vi "Read Mail To Next Actor.vi"(8 "error in (no error)":errorcluster, 11 "Composite Task in":refnum<class "Composite Task.lvclass">) -> (0 "error out":errorcluster, 2 "Mail Strategy.lvclass":refnum<class "Mail Strategy.lvclass">, 3 "Composite Task out":refnum<class "Composite Task.lvclass">)   [LabVIEW 2019, in "Composite Task.lvclass"]
uses:
  Composite Task.lvclass
  Messenger/Mail Strategy/Mail Strategy.lvclass
  Composite Task.lvclass/Composite Task.ctl
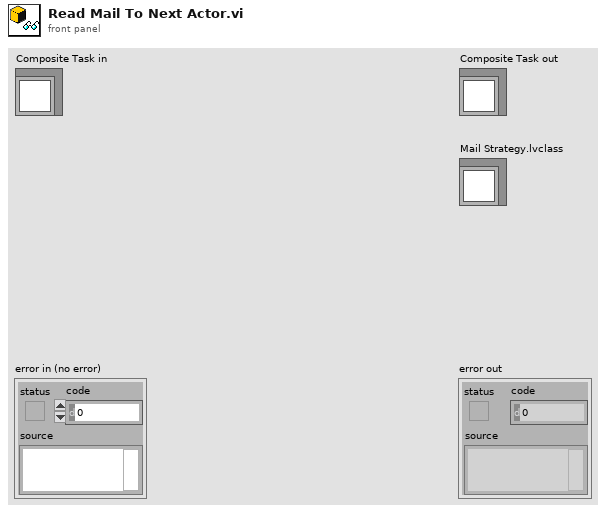
[diagram p1: front panel]
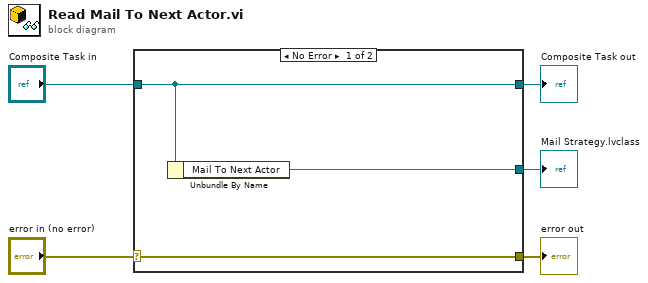
[diagram p0: block diagram]
diagram:
  n1 = case shown="No Error" "error in (no error)" {
    selector: "error in (no error)" -> [w8 w9]
    tunnel: [w8 w9] -> w4
    tunnel: [w7 w10] -> w2
    tunnel: "Composite Task in" -> [w7 w10]
    tunnel: [w6 _] -> w1
    frame No Error {
      n2 = Unbundle By Name(w7) -> ("Mail To Next Actor"=w6:refnum<class "Mail Strategy.lvclass">)
    }
    frame Error {
    }
  }
  "error out" <- w4
  "Composite Task out" <- w2
  "Mail Strategy.lvclass" <- w1
